vi "Interpolate Vsg.vi"(1 "Vsg(B)":cluster{"Vsg":dbl[], "B":dbl[]}, 2 "B":dbl) -> (0 "Vsg":dbl)   [LabVIEW 2016]
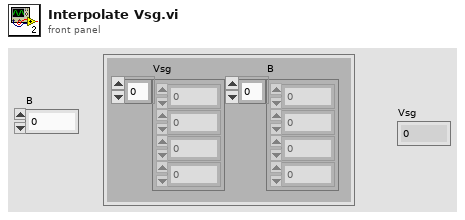
[diagram p1: front panel]
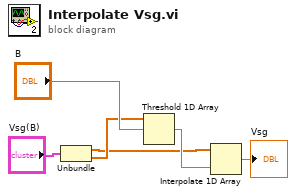
[diagram p0: block diagram]
diagram:
  n1 = Unbundle("Vsg(B)") -> ("Vsg"=w1:dbl[], "B"=w2:dbl[])
  n2 = Threshold 1D Array(2:"B", 3:w2) -> (0:w5:dbl)  [unwired: 1 in]
  n3 = Interpolate 1D Array(1:w5, 2:w1) -> (0:→"Vsg":dbl)
